vi "Calc Tax.vi"(9 "Price":dbl, 10 "Qty":dbl, 11 "Provider":T1) -> (2 "Taxe":dbl)   [LabVIEW 2012]
uses:
  PortFolio-Provider.ctl
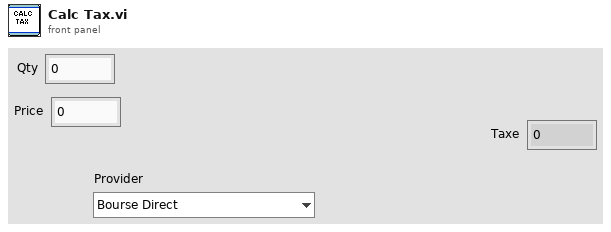
[diagram p1: front panel]
types:
  T1 = typedef "PortFolio-Provider.ctl" = enum16{"Bourse Direct"}
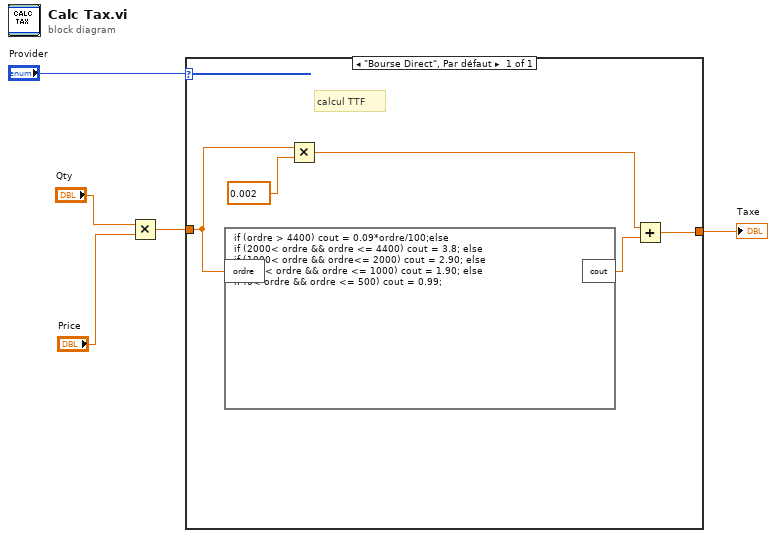
[diagram p0: block diagram]
diagram:
  n1 = Multiply(x="Qty", y="Price") -> (x*y=w2:dbl)
  n2 = case shown="\"Bourse Direct\", Par défaut" "Provider" {
    tunnel: w2 -> [w7]
    tunnel: [w8] -> w1
    frame "Bourse Direct", Default {
      # "calcul TTF"
      n3 = formula code="if (ordre > 4400) cout = 0.09*ordre/100;else\nif (2000< ordre && ordre <= 4400) cout = 3.8; else\nif (1000< ordre && ordre<= 2000) cout = 2.90; else\nif (500< ordre && ordre <= 1000) cout = 1.90; else\nif (0< ordre && ordre <= 500) cout = 0.99;"("ordre"=w7) -> ("cout"=w6:dbl)
      n4 = Multiply(x=w7, y=0.002) -> (x*y=w9:dbl)
      n5 = Add(x=w9, y=w6) -> (x+y=w8:dbl)
    }
  }
  "Taxe" <- w1
